vi "hello world.vi"() -> ()   [LabVIEW 2023]
panel:
  out "String":string="Hello World!"
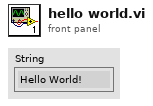
[diagram p1: front panel]
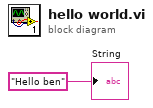
[diagram p0: block diagram]
diagram:
  "String" <- "Hello ben"
